vi "SMO.UI.Basic.TestLauncher.vi"() -> ()   [LabVIEW 2013, in "SMO.UI.Basic.lvclass"]
doc: "JKI State Machine Objects (SMO) 1.0.0.5\nJKI - JKI\nCopyright (c) 2016, JKI"
uses:
  SMO.UI.Basic.lvclass
  <vilib>/JKI/JKI SMO/SMO/SMO.lvclass
  <vilib>/JKI/JKI SMO/SMO.UI/SMO.UI.lvclass
panel:
  out "error out":errorcluster
  in  "Stop":bool
  # "SMO UI Test Launcher"
  # "For instructions on how to use the JKI State Machine Objects, examples and video tutorials, visit:\nhttp://jki.net/state-machine-objects/\n\nJKI State Machine Objects™\nhttp://jki.net/state-machine-objects/\nCopyright (C) 2005-2015, JKI <info@jki.net>\nALL RIGHTS RESERVED"
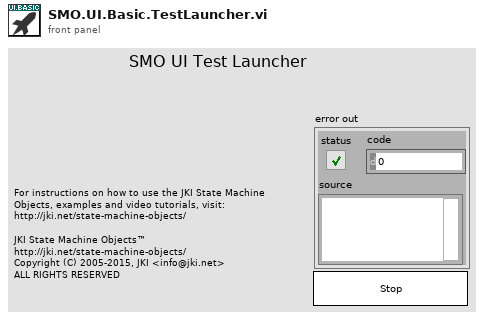
[diagram p1: front panel]
types:
  T1 = cluster{"SMO.UI Public Events":refnum<event-registration>}
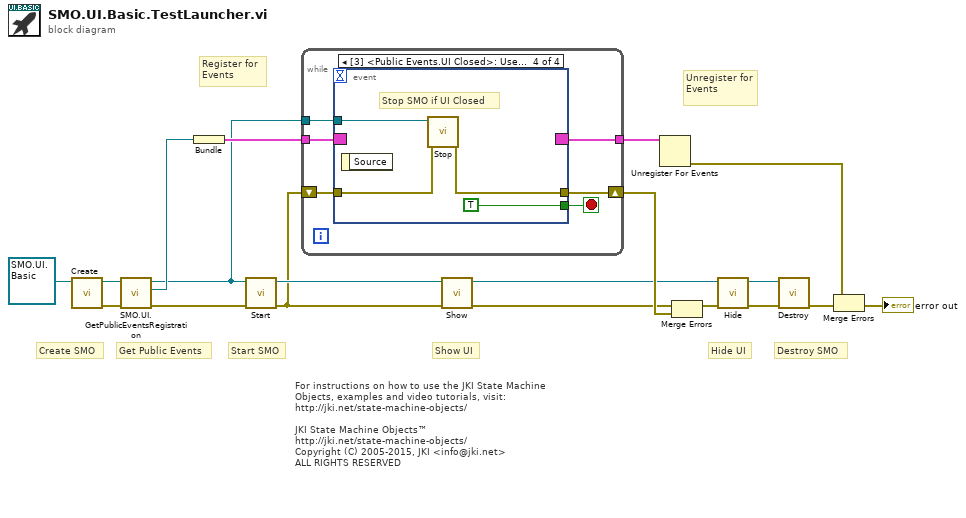
[diagram p0: block diagram]
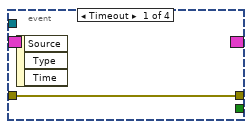
[diagram p2: hidden frame]
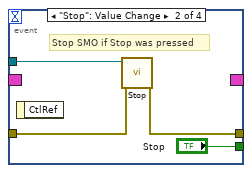
[diagram p3: hidden frame]
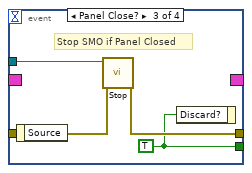
[diagram p4: hidden frame]
diagram:
  # "Hide UI"
  # "Show UI"
  # "For instructions on how to use the JKI State Machine Objects, examples and video tutorials, visit:\nhttp://jki.net/state-machine-objects/\n\nJKI State Machine Objects™\nhttp://jki.net/state-machine-objects/\nCopyright (C) 2005-2015, JKI <info@jki.net>\nALL RIGHTS RESERVED"
  # "Get Public Events"
  # "Start SMO"
  # "Destroy SMO"
  # "Create SMO"
  # "Unregister for Events"
  # "Register for Events"
  n1 = call <vilib>:"Create.vi"("SMO"=refnum<class "SMO.UI.Basic.lvclass"> refnum ("SMO.Template.lvclass")) -> ("error out"=w5:errorcluster, "SMO out"=w4:refnum<class "SMO.UI.Basic.lvclass">)  [unwired: 9 in]
  n2 = call <vilib>:"SMO.UI.GetPublicEventsRegistration.vi"("error in (no error)"=w5, "SMO.UI"=w4) -> ("error out"=w1:errorcluster, "SMO.UI Public Events"=w3:refnum<event-registration>, "SMO.UI out"=w2:refnum<class "SMO.UI.Basic.lvclass">)  [unwired: 7 in]
  n3 = Bundle("SMO.UI Public Events"=w3) -> (w18:T1)  [unwired: 1 in]
  n4 = call <vilib>:"Start.vi"("error in (no error)"=w1, "SMO"=w2) -> ("error out"=w11:errorcluster, "SMO out"=w12:refnum<class "SMO.UI.Basic.lvclass">)  [unwired: 8 in]
  n5 = while {
    shift-right: [w24] -> w17
    shift-left: w11 -> [w23]
    tunnel: w18 -> [w22]
    tunnel: [w21] -> w19
    tunnel: w2 -> [w20]
    stop <- w25 stop-if-true
    n6 = event shown="[3] <Public Events.UI Closed>: User Event" {
      selector: w22 -> [_ _ _ _]
      dyn-events: [_ _ _ _] -> w21
      timeout: _ -> [_ _ _ _]
      tunnel: [_ "Stop" w31 TRUE ("OK")] -> w25
      tunnel: w20 -> [_ w28 w34 w38]
      tunnel: [w26 w29 w33 w37] -> w24
      tunnel: w23 -> [w26 w27 w32 w36]
      event Timeout {
        n7 = event-data() -> ()  [unwired: 1 in, 3 out]
      }
      event "Stop": Value Change {
        # "Stop SMO if Stop was pressed"
        n8 = event-data() -> ()  [unwired: 1 in, 1 out]
        n9 = call <vilib>:"Stop.vi"("error in (no error)"=w27, "SMO"=w28) -> ("error out"=w29:errorcluster)  [unwired: 8 in, 1 out]
      }
      event Panel Close? {
        w31 = TRUE ("OK")
        # "Stop SMO if Panel Closed"
        n10 = event-data() -> ()  [unwired: 1 in, 1 out]
        n11 = call <vilib>:"Stop.vi"("error in (no error)"=w32, "SMO"=w34) -> ("error out"=w33:errorcluster)  [unwired: 8 in, 1 out]
        n12 = event-data("Discard?"=w31) -> ()  [unwired: 1 in, 1 out]
      }
      event User Event {
        # "Stop SMO if UI Closed"
        n13 = event-data() -> ()  [unwired: 1 in, 1 out]
        n14 = call <vilib>:"Stop.vi"("error in (no error)"=w36, "SMO"=w38) -> ("error out"=w37:errorcluster)  [unwired: 8 in, 1 out]
      }
    }
  }
  n15 = call <vilib>:"Show.vi"("error in (no error)"=w11, "SMO.UI"=w12) -> ("error out"=w10:errorcluster, "SMO.UI out"=w9:refnum<class "SMO.UI.Basic.lvclass">)  [unwired: 8 in]
  n16 = Unregister For Events(event registration refnum=w19) -> (error out=w16:errorcluster)  [unwired: 1 in]
  n17 = Merge Errors(w10, w17) -> (w7:errorcluster)
  n18 = call <vilib>:"Hide.vi"("error in (no error)"=w7, "SMO.UI"=w9) -> ("error out"=w6:errorcluster, "SMO.UI out"=w8:refnum<class "SMO.UI.Basic.lvclass">)  [unwired: 8 in]
  n19 = call <vilib>:"Destroy.vi"("error in (no error)"=w6, "SMO"=w8) -> ("error out"=w14:errorcluster)  [unwired: 9 in]
  n20 = Merge Errors(w16, w14) -> (→"error out":errorcluster)
